vi "AerotechGetTarget.vi"(0 "error in (no error)":errorcluster) -> (3 "error out":errorcluster, 5 "AEROTECH.TARGET":T1)   [LabVIEW 2009]
uses:
  Controls/AerotechTarget.ctl
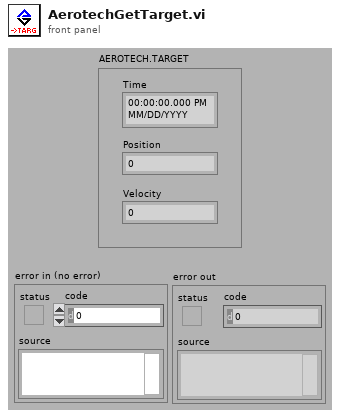
[diagram p1: front panel]
types:
  T1 = typedef "AerotechTarget.ctl" = cluster{"Time":timestamp, "Position":dbl, "Velocity":dbl}
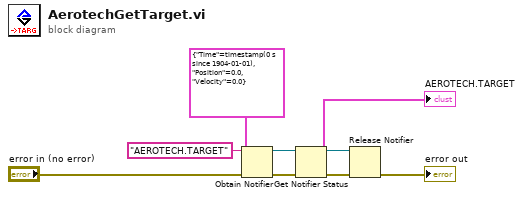
[diagram p0: block diagram]
diagram:
  n1 = Obtain Notifier(name (unnamed)="AEROTECH.TARGET", notification data type=T1 {"Time"=timestamp(0 s since 1904-01-01), "Position"=0.0, "Velocity"=0.0} ("AEROTECH.TARGET"), error in (no error)="error in (no error)") -> (notifier out=w7:refnum<notifier>, error out=w8:errorcluster)  [unwired: 1 in, 1 out]
  n2 = Get Notifier Status(notifier=w7, error in (no error)=w8) -> (notifier out=w5:refnum<notifier>, current notification=→"AEROTECH.TARGET":T1, error out=w6:errorcluster)  [unwired: 2 out]
  n3 = Release Notifier(notifier=w5, error in (no error)=w6) -> (error out=→"error out":errorcluster)  [unwired: 1 in, 2 out]
